vi "Draw Trajectory.vi"(0 "Picture in":refnum<vi>, 1 "Robot Index":i32, 5 "Trajectory Data":T3, 7 "time":dbl, 9 "new picture in":picture, 10 "MEGA?":bool, 11 "Hide Path":bool, 12 "MEGA traj":T2 {"?"."Limits"."StoopidFast (fps)" min=0.0; "?"."Limits"."Jerk (fps^3)" min=0.0 step=1.0; "?"."Limits"."Accel (fps^2)" min=0.0; "?"."Limits"."Velocity (fps)" min=0.0; "?"."Overrides"."Angle Override" step=5.0; "?"."Overrides"."Velocity Override" step=5.0; "?"."Overrides"."Angular Override" step=5.0; "?"."Angular Limits"."Jerk (deg/s^3)" min=0.0 step=1.0; "?"."Angular Limits"."Accel (deg/s^2)" min=0.0; "?"."Angular Limits"."Velocity (deg/s)" min=0.0}) -> (3 "Path Points MEGA":cluster{"x":dbl, "y":dbl}[][](array[cluster]), 4 "new picture":picture, 6 "Output Point":T12, 14 "Output Point MEGA":T1(array[cluster]), 15 "Path Points":cluster{"x":dbl, "y":dbl}[](array[cluster]))   [LabVIEW 2023]
uses:
  Types/Trajectory Data.ctl
  Types/Segment Type.ctl
  FileIO/MEGA traj.ctl
  Types/Single Cmd Info.ctl
  <vilib>/picture/picture.llb/imagedata.ctl
  Types/Limits.ctl
  Types/Overrides.ctl
  Types/Angluar Limits.ctl
  Types/Drive Type.ctl
  Types/Path Type.ctl
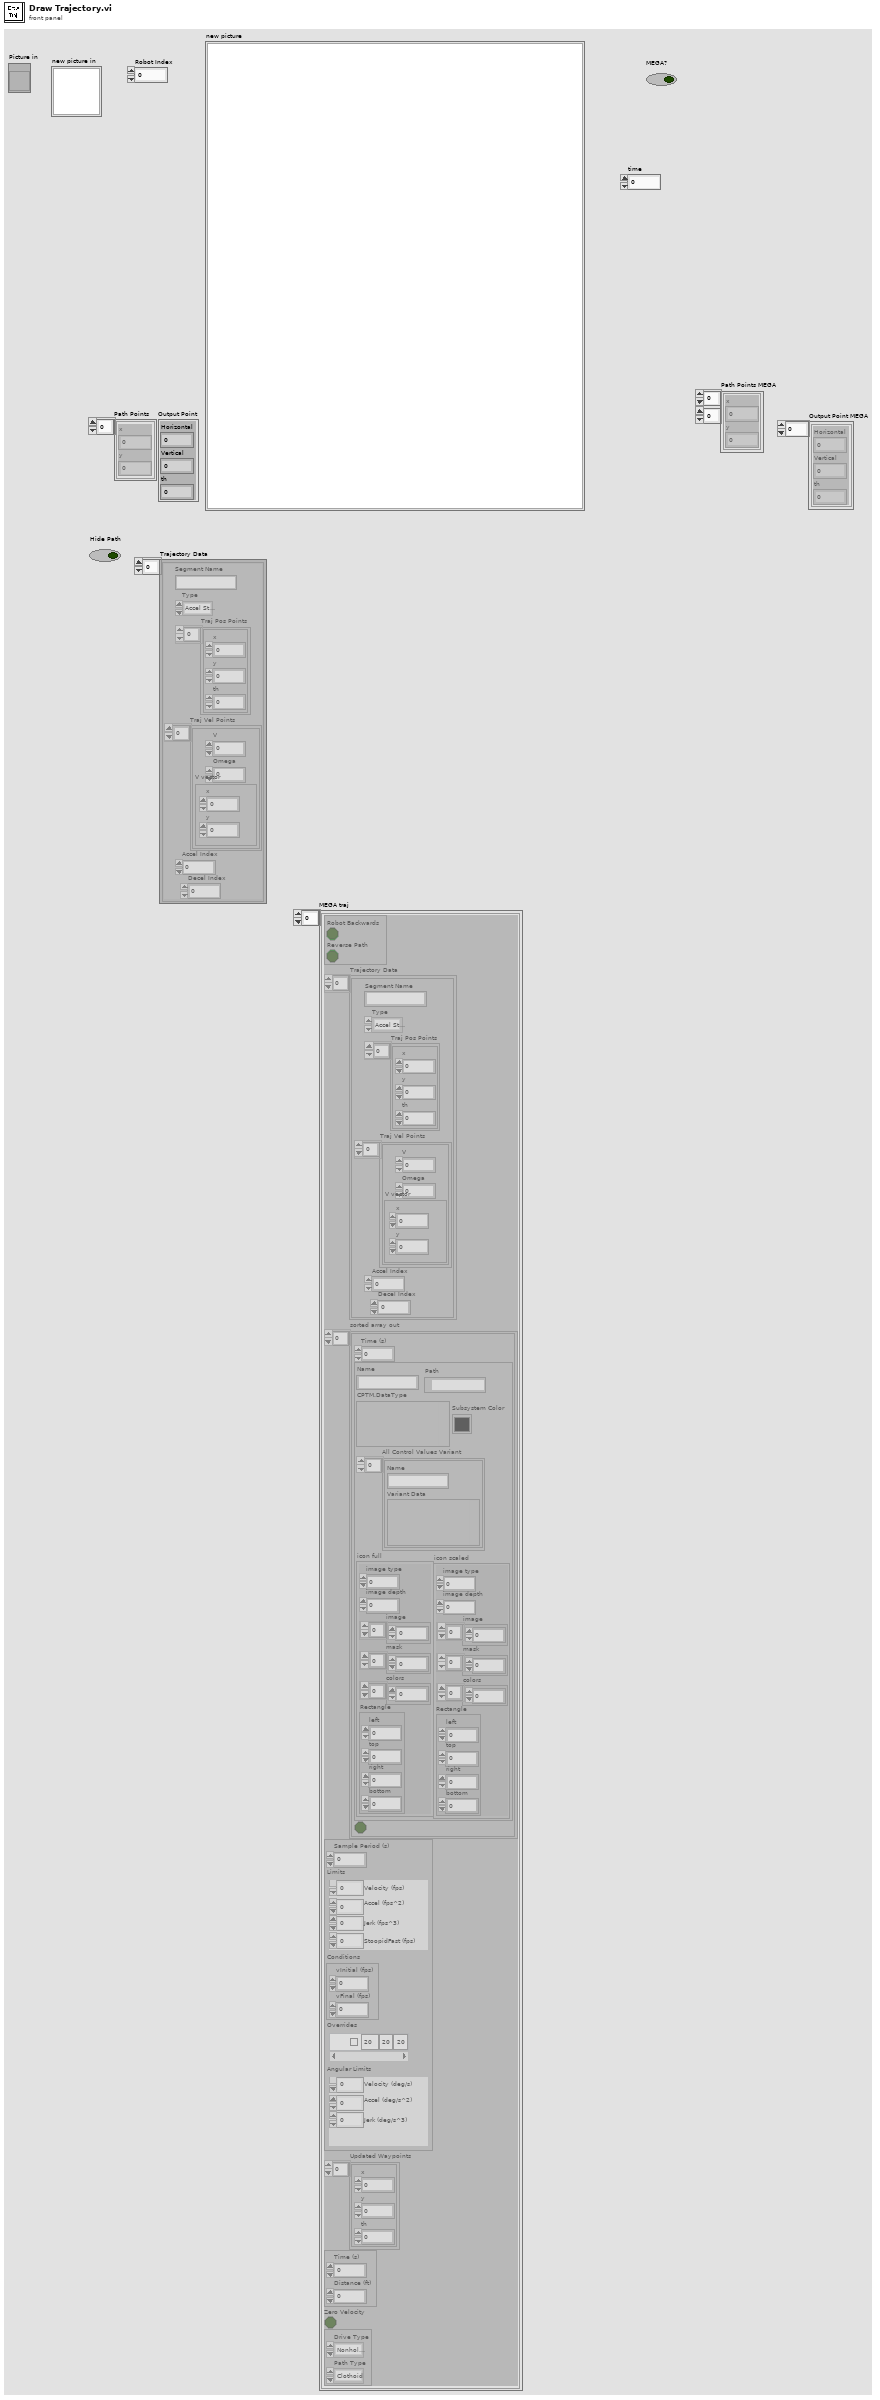
[diagram p1: front panel]
types:
  T1 = cluster{"Horizontal":dbl, "Vertical":dbl, "th":dbl}[]
  T2 = typedef "MEGA traj.ctl" = cluster{cluster{"Robot Backwards":bool, "Reverse Path":bool}, "Trajectory Data":T3, "sorted array out":cluster{"Time (s)":dbl, T5, bool}[], cluster{"Sample Period (s)":dbl, "Limits":T7, "Conditions":cluster{"vInitial (fps)":dbl, "vFinal (fps)":dbl}, "Overrides":T8, "Angular Limits":T9}, "Updated Waypoints":cluster{"x":dbl, "y":dbl, "th":dbl}[], cluster{"Time (s)":dbl, "Distance (ft)":dbl}, "Zero Velocity":bool, cluster{"Drive Type":T10, "Path Type":T11}}[]
  T3 = typedef "Trajectory Data.ctl" = cluster{"Segment Name":string, "Type":T4, "Traj Pos Points":cluster{"x":dbl, "y":dbl, "th":dbl}[], "Traj Vel Points":cluster{"V":dbl, "Omega":dbl, "V vector":cluster{"y":dbl, "x":dbl}}[], "Accel Index":i32, "Decel Index":i32}[]
  T4 = typedef "Segment Type.ctl" = enum16{"Accel Straight", "Const Straight", "Blend", "Circle", "Bezier"}
  T5 = typedef "Single Cmd Info.ctl" = cluster{"Name":string, "CPTM.DataType":variant, "All Control Values Variant":cluster{"Name":string, "Variant Data":variant}[], "icon full":T6, "icon scaled":T6, "Path":path, "Subsystem Color":u32}
  T6 = typedef "imagedata.ctl" = cluster{"image type":i32, "image depth":i32, "image":u8[], "mask":u8[], "colors":u32[], "Rectangle":cluster{"left":i16, "top":i16, "right":i16, "bottom":i16}}
  T7 = typedef "Limits.ctl" = cluster{"Velocity (fps)":dbl, "Accel (fps^2)":dbl, "Jerk (fps^3)":dbl, "StoopidFast (fps)":dbl}
  T8 = typedef "Overrides.ctl" = cluster{"Count":string, "Angular Override":dbl, "Enabled?":bool, "Velocity Override":dbl, "Angle Override":dbl}[]
  T9 = typedef "Angluar Limits.ctl" = cluster{"Velocity (deg/s)":dbl, "Accel (deg/s^2)":dbl, "Jerk (deg/s^3)":dbl}
  T10 = typedef "Drive Type.ctl" = enum16{"Nonholonomic", "Holonomic"}
  T11 = typedef "Path Type.ctl" = enum16{"Clothoid", "Bezier"}
  T12 = cluster{"Horizontal":dbl, "Vertical":dbl, "th":dbl}
  T13 = cluster{"Width":u16, "Style":enum32{"Solid", "Dash", "Dot", "DashDot", "DashDotDot"}}
  T14 = typedef "LVPositionTypeDef.ctl" = cluster{"Left":i32, "Top":i32}
  T15 = typedef "LVBoundsTypeDef.ctl" = cluster{"Width":u32, "Height":u32}
  T16 = cluster{"V":dbl, "Omega":dbl, "V vector":cluster{"y":dbl, "x":dbl}}[]
  T17 = cluster{cluster{"Robot Backwards":bool, "Reverse Path":bool}, "Trajectory Data":T3, "sorted array out":cluster{"Time (s)":dbl, T5, bool}[], cluster{"Sample Period (s)":dbl, "Limits":T7, "Conditions":cluster{"vInitial (fps)":dbl, "vFinal (fps)":dbl}, "Overrides":T8, "Angular Limits":T9}, "Updated Waypoints":cluster{"x":dbl, "y":dbl, "th":dbl}[], cluster{"Time (s)":dbl, "Distance (ft)":dbl}, "Zero Velocity":bool, cluster{"Drive Type":T10, "Path Type":T11}}
  T18 = cluster{"Robot Backwards":bool, "Reverse Path":bool}
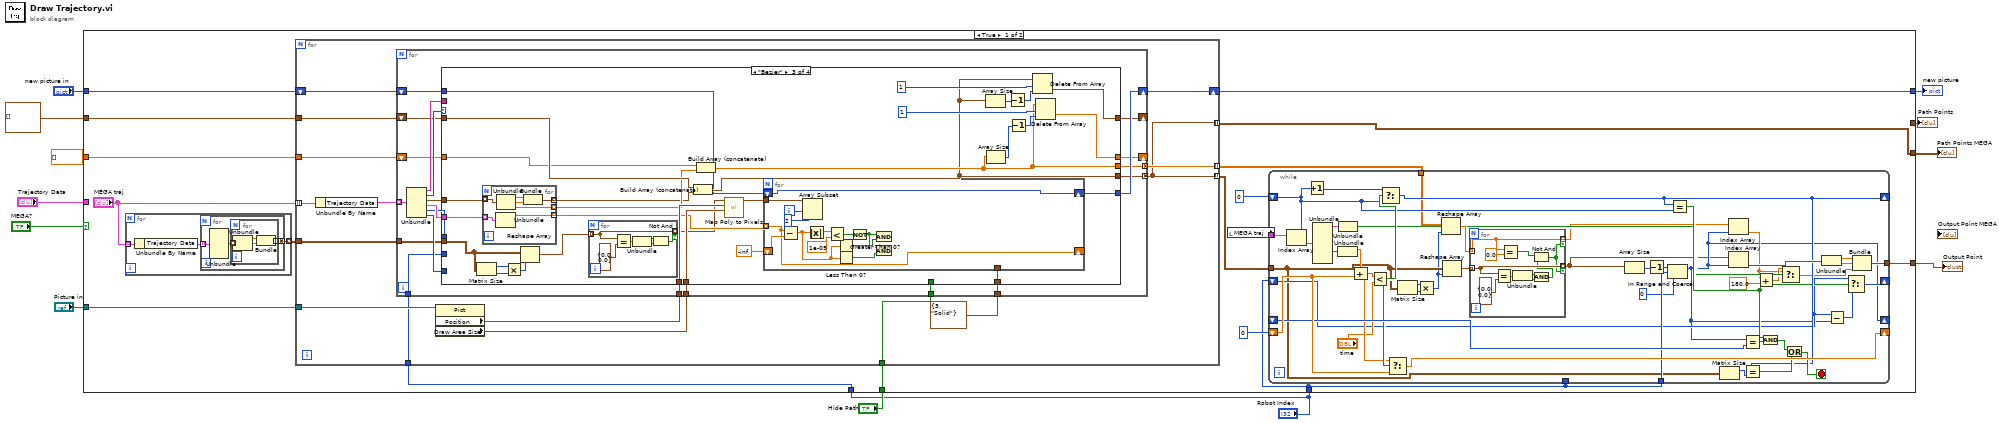
[diagram p0: block diagram]
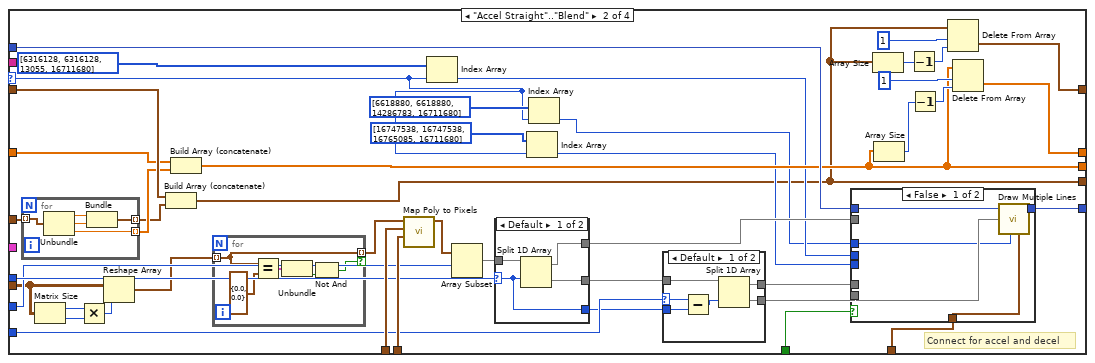
[diagram p3: hidden frame]
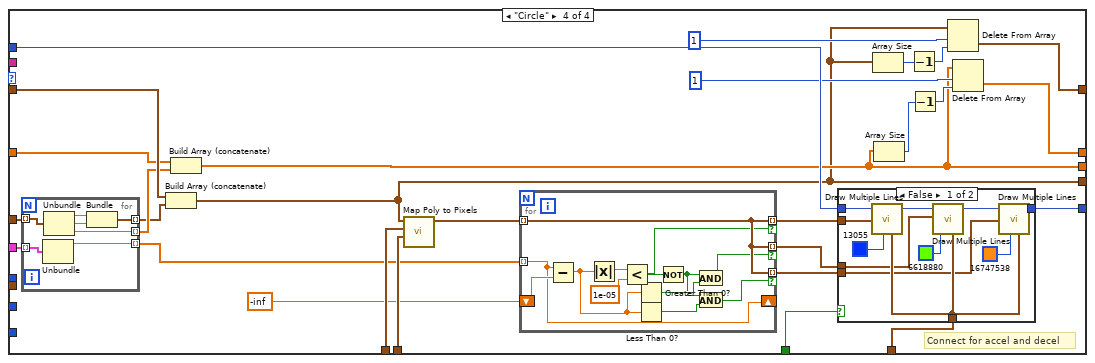
[diagram p7: hidden frame]
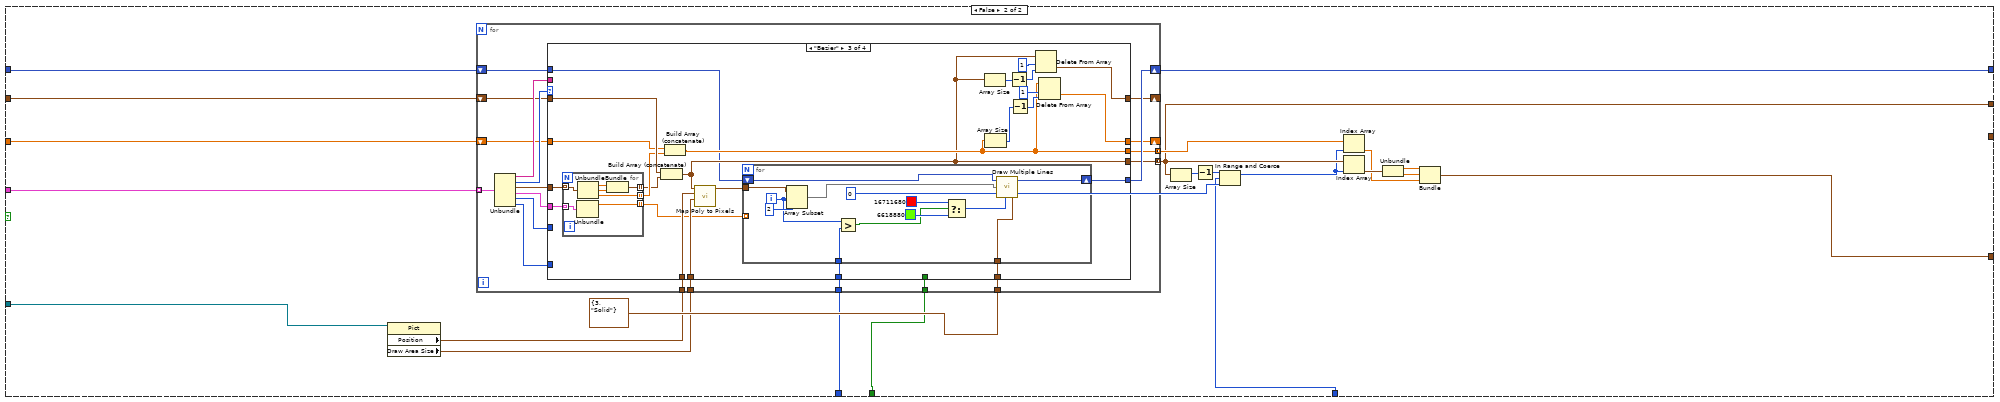
[diagram p9: hidden frame]
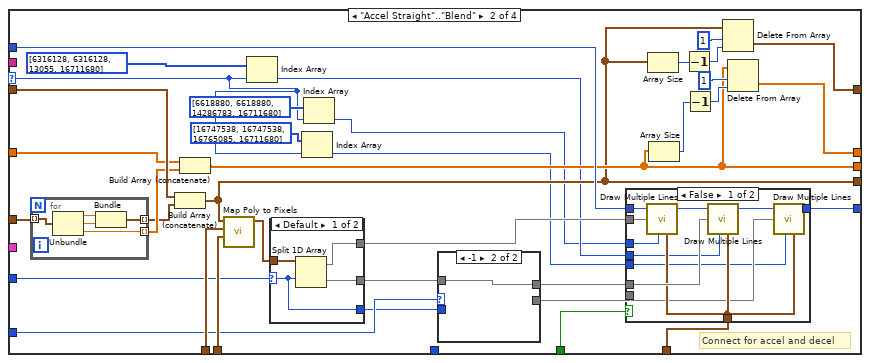
[diagram p11: hidden frame]
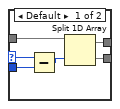
[diagram p13: hidden frame]
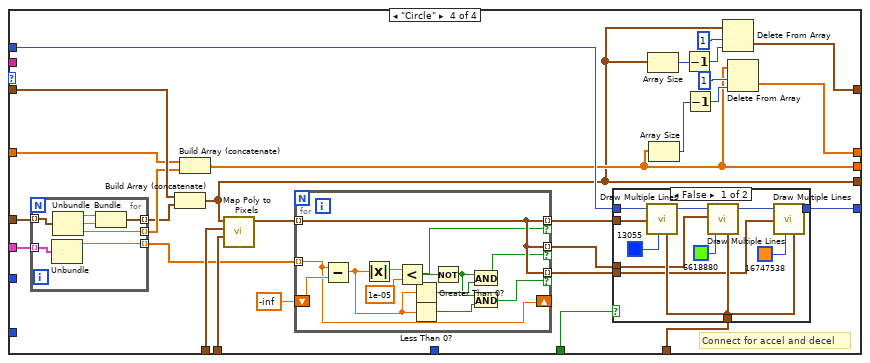
[diagram p15: hidden frame]
diagram:
  n1 = case shown="True" "MEGA?" {
    tunnel: "Picture in" -> [w29 w345]
    tunnel: "new picture in" -> [w28 w344]
    tunnel: [w27 w340] -> w10
    tunnel: [_ w334] -> w9
    tunnel: cluster{"x":dbl, "y":dbl}[] [] -> [w26 w329]
    tunnel: dbl[] [] -> [w25 w328]
    tunnel: "Trajectory Data" -> [_ w327]
    tunnel: "Hide Path" -> [w24 w326]
    tunnel: [w17 _] -> w3
    tunnel: "Robot Index" -> [w16 w325]
    tunnel: [w21 w324] -> w2
    tunnel: "Robot Index" -> [w15 w323]
    frame True {
      n2 = for {
        tunnel: "MEGA traj" -> [w32] mode=indexing
        tunnel: [w30] -> w13 mode=indexing
        n3 = Unbundle By Name(w32) -> ("Trajectory Data"=w31:T3)
        n4 = for {
          tunnel: w31 -> [w35] mode=indexing
          tunnel: [w33] -> w30 mode=concatenating
          n5 = Unbundle(w35) -> ("Traj Pos Points"=w34:cluster{"x":dbl, "y":dbl, "th":dbl}[])  [unwired: 5 out]
          n6 = for {
            tunnel: w34 -> [w37] mode=indexing
            tunnel: [w36] -> w33 mode=indexing
            n7 = Unbundle(w37) -> ("x"=w39:dbl, "y"=w38:dbl)  [unwired: 1 out]
            n8 = Bundle("x"=w39, "y"=w38) -> (w36:cluster{"x":dbl, "y":dbl})  [unwired: 1 in]
          }
        }
      }
      n9 = for {
        tunnel: w29 -> [w110]
        tunnel: [w99] -> w17 mode=indexing
        tunnel: w26 -> [w104]
        tunnel: w25 -> [w103]
        shift-right: [w105] -> w27
        shift-left: w28 -> [w109]
        tunnel: w24 -> [w102]
        tunnel: "MEGA traj" -> [w97] mode=indexing
        tunnel: [w100] -> w18 mode=indexing
        tunnel: [w99] -> w19 mode=indexing
        tunnel: w15 -> [w98]
        tunnel: w13 -> [w96]
        n10 = Unbundle By Name(w97) -> ("Trajectory Data"=w101:T3)
        n11 = property on="Property Node" class="Pict"(reference=w110) -> ("Position"=w106:T14, "Draw Area Size"=w107:T15)  [unwired: 1 in, 2 out]
        n12 = for {
          tunnel: w101 -> [w131] mode=indexing
          shift-right: [w125] -> w105
          shift-left: w109 -> [w124]
          tunnel: T13 {"Width"=3, "Style"=enum."Solid"} ("pen") -> [w128]
          tunnel: w107 -> [w127]
          tunnel: w106 -> [w126]
          tunnel: [w122] -> w99 mode=concatenating
          tunnel: [w121] -> w100 mode=concatenating
          shift-right: [w120] -> _
          shift-left: w104 -> [w119]
          shift-right: [w118] -> _
          shift-left: w103 -> [w117]
          tunnel: w102 -> [w115]
          tunnel: w98 -> [w112]
          tunnel: w96 -> [w111]
          n13 = Unbundle(w131) -> ("Segment Name"=w130:string, "Type"=w123:T4, "Traj Pos Points"=w113:cluster{"x":dbl, "y":dbl, "th":dbl}[], "Traj Vel Points"=w129:T16, "Accel Index"=w114:i32, "Decel Index"=w116:i32)
          n14 = case shown="\"Bezier\"" w123 {
            selector: w123 -> [_ w148 _ _]
            tunnel: w130 -> [_ _ _ _]
            tunnel: w113 -> [_ w178 w237 w291]
            tunnel: w129 -> [_ _ w220 w270]
            tunnel: w128 -> [_ w157 w217 w274]
            tunnel: w127 -> [_ w177 w236 w290]
            tunnel: w126 -> [_ w175 w235 w288]
            tunnel: [w134 w158 w215 w275] -> w125
            tunnel: w124 -> [w134 w176 w216 w289]
            tunnel: [_ w142 w221 w272] -> w122
            tunnel: [_ w164 w225 w278] -> w121
            tunnel: w114 -> [_ w161 _ _]
            tunnel: [w133 w169 w230 w283] -> w120
            tunnel: w119 -> [w133 w172 w233 w286]
            tunnel: [w132 w165 w226 w279] -> w118
            tunnel: w117 -> [w132 w162 w223 w276]
            tunnel: w116 -> [_ w160 _ _]
            tunnel: w115 -> [_ w145 _ w271]
            tunnel: w112 -> [_ w141 _ _]
            tunnel: w111 -> [_ w140 w210 _]
            frame Default {
            }
            frame "Accel Straight".."Blend" {
              # "Connect for accel and decel"
              n15 = for {
                tunnel: w178 -> [w207] mode=indexing
                tunnel: [w206] -> w153 mode=indexing
                tunnel: [w203] -> w163 mode=indexing
                n16 = Unbundle(w207) -> ("x"=w205:dbl, "y"=w204:dbl, "th"=w203:dbl)
                n17 = Bundle("x"=w205, "y"=w204) -> (w206:cluster{"x":dbl, "y":dbl})  [unwired: 1 in]
              }
              n18 = Matrix Size(0:w140) -> (1:w139:i32, 2:w138:i32)
              n19 = Multiply(x=w139, y=w138) -> (x*y=w137:i32)
              n20 = Reshape Array(w140, w137) -> (w136:cluster{"x":dbl, "y":dbl}[])
              n21 = Build Array (concatenate)(w172, w153) -> (w142:cluster{"x":dbl, "y":dbl}[])
              n22 = Build Array (concatenate)(w162, w163) -> (w164:dbl[])
              n23 = for {
                tunnel: w136 -> [w184] mode=indexing
                tunnel: [w184] -> w135 mode=indexing if=w179
                n24 = Equal?(x=w184, y=cluster{"x":dbl, "y":dbl} {"x"=0.0, "y"=0.0}) -> (x = y?=w182:cluster{"x":bool, "y":bool})
                n25 = Unbundle(w182) -> ("x"=w180:bool, "y"=w181:bool)
                n26 = Not And(1:w181, 2:w180) -> (0:w179:bool)
              }
              n27 = call "Map Poly to Pixels.vi"("Draw Area Size"=w177, "Position"=w175, "Coords"=w135) -> ("Coords"=w143:cluster{"Horizontal":dbl, "Vertical":dbl}[])  [unwired: 8 in]
              n28 = Index Array(array=u32[] [6316128, 6316128, 13055, 16711680], index=w148) -> (element=w151:u32)
              n29 = Array Subset(array=w143, index=w141) -> (w144:cluster{"Horizontal":dbl, "Vertical":dbl}[])  [unwired: 1 in]
              n30 = case shown="Default" w161 {
                selector: w161 -> [w198 _]
                tunnel: w144 -> [w201 w202]
                tunnel: [w199 _] -> w152
                tunnel: [w200 w202] -> w155
                tunnel: [w198 _] -> w154
                frame Default {
                  n31 = Split 1D Array(array=w201, index=w198) -> (first subarray=w199:cluster{"Horizontal":dbl, "Vertical":dbl}[], second subarray=w200:cluster{"Horizontal":dbl, "Vertical":dbl}[])
                }
                frame -1 {
                }
              }
              n32 = Index Array(array=u32[] [16747538, 16747538, 16765085, 16711680], index=w148) -> (element=w146:u32)
              n33 = Index Array(array=u32[] [6618880, 6618880, 14286783, 16711680], index=w148) -> (element=w147:u32)
              n34 = case shown="Default" w160 {
                selector: w160 -> [w193 _]
                tunnel: w155 -> [w196 w197]
                tunnel: [w195 w197] -> w159
                tunnel: [w194 _] -> w156
                tunnel: w154 -> [w192 _]
                frame Default {
                  n35 = Subtract(x=w193, y=w192) -> (x-y=w191:i32)
                  n36 = Split 1D Array(array=w196, index=w191) -> (first subarray=w195:cluster{"Horizontal":dbl, "Vertical":dbl}[], second subarray=w194:cluster{"Horizontal":dbl, "Vertical":dbl}[])
                }
                frame -1 {
                }
              }
              n37 = case shown="False" w145 {
                tunnel: w176 -> [w186 w190]
                tunnel: w159 -> [_ _]
                tunnel: [w189 w190] -> w158
                tunnel: w157 -> [w188 _]
                tunnel: w156 -> [w187 _]
                tunnel: w152 -> [_ _]
                tunnel: w151 -> [_ _]
                tunnel: w147 -> [w185 _]
                tunnel: w146 -> [_ _]
                frame False {
                  n38 = call <vilib>:"Draw Multiple Lines.vi"("picture"=w186, "line endpoints"=w187, "color(black)"=w185, "pen"=w188) -> ("new picture"=w189:picture)  [unwired: 5 in]
                }
                frame True {
                }
              }
              n39 = Array Size(array=w142) -> (size(s)=w173:i32)
              n40 = Array Size(array=w164) -> (size(s)=w166:i32)
              n41 = Decrement(x=w173) -> (x-1=w170:i32)
              n42 = Decrement(x=w166) -> (x-1=w168:i32)
              n43 = Delete From Array(array=w142, length=1, index=w170) -> (deleted portion=w169:cluster{"x":dbl, "y":dbl}[])  [unwired: 1 out]
              n44 = Delete From Array(array=w164, length=1, index=w168) -> (deleted portion=w165:dbl[])  [unwired: 1 out]
            }
            frame "Bezier" {
              n45 = Matrix Size(0:w210) -> (1:w209:i32, 2:w213:i32)
              n46 = for {
                tunnel: w237 -> [w263] mode=indexing
                tunnel: [w262] -> w222 mode=indexing
                tunnel: [w259] -> w224 mode=indexing
                tunnel: w220 -> [w258] mode=indexing
                tunnel: [w257] -> w219 mode=indexing
                n47 = Unbundle(w258) -> ("V"=w257:dbl)  [unwired: 2 out]
                n48 = Unbundle(w263) -> ("x"=w261:dbl, "y"=w260:dbl, "th"=w259:dbl)
                n49 = Bundle("x"=w261, "y"=w260) -> (w262:cluster{"x":dbl, "y":dbl})  [unwired: 1 in]
              }
              n50 = Multiply(x=w209, y=w213) -> (x*y=w212:i32)
              n51 = Reshape Array(w210, w212) -> (w211:cluster{"x":dbl, "y":dbl}[])
              n52 = for {
                tunnel: w211 -> [w243] mode=indexing
                tunnel: [w243] -> w208 mode=indexing if=w238
                n53 = Equal?(x=w243, y=cluster{"x":dbl, "y":dbl} {"x"=0.0, "y"=0.0}) -> (x = y?=w241:cluster{"x":bool, "y":bool})
                n54 = Unbundle(w241) -> ("x"=w239:bool, "y"=w240:bool)
                n55 = Not And(1:w240, 2:w239) -> (0:w238:bool)
              }
              n56 = Build Array (concatenate)(w233, w222) -> (w221:cluster{"x":dbl, "y":dbl}[])
              n57 = Build Array (concatenate)(w223, w224) -> (w225:dbl[])
              n58 = call "Map Poly to Pixels.vi"("Draw Area Size"=w236, "Position"=w235, "Coords"=w208) -> ("Coords"=w214:cluster{"Horizontal":dbl, "Vertical":dbl}[])  [unwired: 8 in]
              n59 = for {
                tunnel: w214 -> [w245]
                tunnel: w219 -> [w253] mode=indexing
                shift-right: [w253] -> _
                shift-left: -inf -> [w256]
                tunnel: w217 -> [_]
                shift-right: [w244] -> w215
                shift-left: w216 -> [w244]
                i -> [w247]
                n60 = Subtract(x=w253, y=w256) -> (x-y=w251:dbl)
                n61 = Array Subset(array=w245, index=w247, length=2) -> ()  [unwired: 1 out]
                n62 = Absolute Value(x=w251) -> (abs(x)=w255:dbl)
                n63 = Less?(x=w255, y=1e-05) -> (x < y?=w248:bool)
                n64 = Greater Than 0?(x=w251) -> (x > 0?=w252:bool)
                n65 = Less Than 0?(x=w251) -> (x < 0?=w250:bool)
                n66 = Not(x=w248) -> (.not. x?=w249:bool)
                n67 = And(x=w249, y=w252) -> ()  [unwired: 1 out]
                n68 = And(x=w249, y=w250) -> ()  [unwired: 1 out]
              }
              n69 = Array Size(array=w221) -> (size(s)=w234:i32)
              n70 = Array Size(array=w225) -> (size(s)=w227:i32)
              n71 = Decrement(x=w234) -> (x-1=w231:i32)
              n72 = Decrement(x=w227) -> (x-1=w229:i32)
              n73 = Delete From Array(array=w221, length=1, index=w231) -> (deleted portion=w230:cluster{"x":dbl, "y":dbl}[])  [unwired: 1 out]
              n74 = Delete From Array(array=w225, length=1, index=w229) -> (deleted portion=w226:dbl[])  [unwired: 1 out]
            }
            frame "Circle" {
              # "Connect for accel and decel"
              n75 = for {
                tunnel: w291 -> [w322] mode=indexing
                tunnel: [w321] -> w273 mode=indexing
                tunnel: [w318] -> w277 mode=indexing
                tunnel: w270 -> [w317] mode=indexing
                tunnel: [w316] -> w269 mode=indexing
                n76 = Unbundle(w317) -> ("V"=w316:dbl)  [unwired: 2 out]
                n77 = Unbundle(w322) -> ("x"=w320:dbl, "y"=w319:dbl, "th"=w318:dbl)
                n78 = Bundle("x"=w320, "y"=w319) -> (w321:cluster{"x":dbl, "y":dbl})  [unwired: 1 in]
              }
              n79 = Build Array (concatenate)(w286, w273) -> (w272:cluster{"x":dbl, "y":dbl}[])
              n80 = Build Array (concatenate)(w276, w277) -> (w278:dbl[])
              n81 = call "Map Poly to Pixels.vi"("Draw Area Size"=w290, "Position"=w288, "Coords"=w272) -> ("Coords"=w264:cluster{"Horizontal":dbl, "Vertical":dbl}[])  [unwired: 8 in]
              n82 = for {
                tunnel: w264 -> [w300] mode=indexing
                tunnel: w269 -> [w299] mode=indexing
                shift-right: [w299] -> _
                shift-left: -inf -> [w303]
                tunnel: [w300] -> w267 mode=indexing if=w294
                tunnel: [w300] -> w266 mode=indexing if=w293
                tunnel: [w300] -> w265 mode=indexing if=w292
                n83 = Subtract(x=w299, y=w303) -> (x-y=w297:dbl)
                n84 = Absolute Value(x=w297) -> (abs(x)=w302:dbl)
                n85 = Less?(x=w302, y=1e-05) -> (x < y?=w294:bool)
                n86 = Greater Than 0?(x=w297) -> (x > 0?=w298:bool)
                n87 = Less Than 0?(x=w297) -> (x < 0?=w296:bool)
                n88 = Not(x=w294) -> (.not. x?=w295:bool)
                n89 = And(x=w295, y=w298) -> (x .and. y?=w293:bool)
                n90 = And(x=w295, y=w296) -> (x .and. y?=w292:bool)
              }
              n91 = case shown="False" w271 {
                tunnel: w289 -> [w314 w315]
                tunnel: [w311 w315] -> w275
                tunnel: w274 -> [w310 _]
                tunnel: w267 -> [w307 _]
                tunnel: w266 -> [w306 _]
                tunnel: w265 -> [w305 _]
                frame False {
                  n92 = call <vilib>:"Draw Multiple Lines.vi"("picture"=w314, "line endpoints"=w307, "color(black)"=u32 13055, "pen"=w310) -> ("new picture"=w313:picture)  [unwired: 5 in]
                  n93 = call <vilib>:"Draw Multiple Lines.vi"("picture"=w313, "line endpoints"=w306, "color(black)"=u32 6618880, "pen"=w310) -> ("new picture"=w312:picture)  [unwired: 5 in]
                  n94 = call <vilib>:"Draw Multiple Lines.vi"("picture"=w312, "line endpoints"=w305, "color(black)"=u32 16747538, "pen"=w310) -> ("new picture"=w311:picture)  [unwired: 5 in]
                }
                frame True {
                }
              }
              n95 = Array Size(array=w272) -> (size(s)=w287:i32)
              n96 = Array Size(array=w278) -> (size(s)=w280:i32)
              n97 = Decrement(x=w287) -> (x-1=w284:i32)
              n98 = Decrement(x=w280) -> (x-1=w282:i32)
              n99 = Delete From Array(array=w272, length=1, index=w284) -> (deleted portion=w283:cluster{"x":dbl, "y":dbl}[])  [unwired: 1 out]
              n100 = Delete From Array(array=w278, length=1, index=w282) -> (deleted portion=w279:dbl[])  [unwired: 1 out]
            }
          }
        }
      }
      n101 = local read "MEGA traj"() -> (w23:T2)
      n102 = while {
        tunnel: w16 -> [w61]
        tunnel: w19 -> [w56]
        tunnel: w18 -> [w57]
        shift-right: [w66] -> _
        shift-left: 0 -> [w65]
        tunnel: w23 -> [w84]
        shift-right: [w79] -> _
        shift-left: 0 -> [w80]
        shift-right: [w42] -> _
        shift-left: _ -> [w72]
        shift-right: [w64] -> _
        shift-left: w16 -> [w60]
        tunnel: [w50] -> w21
        tunnel: w16 -> [_]
        stop <- w73 stop-if-true
        n103 = Index Array(array=w84, index=w65) -> (element=w83:T17)
        n104 = Increment(x=w65) -> (x+1=w85:i32)
        n105 = Unbundle(w83) -> (w48:T18, w82:cluster{"Time (s)":dbl, "Distance (ft)":dbl})  [unwired: 6 out]
        n106 = Unbundle(w82) -> ("Time (s)"=w81:dbl)  [unwired: 1 out]
        n107 = Unbundle(w48) -> ("Robot Backwards"=w47:bool)  [unwired: 1 out]
        n108 = Add(x=w81, y=w80) -> (x+y=w70:dbl)
        n109 = Less?(x=w70, y="time") -> (x < y?=w71:bool)
        n110 = Select(t=w85, s=w71, f=w65) -> (s? t:f=w66:i32)
        n111 = Select(t=w70, s=w71, f=w80) -> (s? t:f=w79:dbl)
        n112 = Matrix Size(0:w56) -> (1:w55:i32, 2:w54:i32)
        n113 = Multiply(x=w55, y=w54) -> (x*y=w53:i32)
        n114 = Reshape Array(w57, w53) -> (w51:dbl[])
        n115 = Reshape Array(w56, w53) -> (w52:cluster{"x":dbl, "y":dbl}[])
        n116 = for {
          tunnel: w52 -> [w95] mode=indexing
          tunnel: [w95] -> w40 mode=indexing if=w88
          tunnel: w51 -> [w92] mode=indexing
          tunnel: [w92] -> w41 mode=indexing if=w88
          n117 = Equal?(x=w95, y=cluster{"x":dbl, "y":dbl} {"x"=0.0, "y"=0.0}) -> (x = y?=w93:cluster{"x":bool, "y":bool})
          n118 = Equal?(x=w92, y=0.0) -> (x = y?=w86:bool)
          n119 = Unbundle(w93) -> ("x"=w89:bool, "y"=w90:bool)
          n120 = And(x=w89, y=w90) -> (x .and. y?=w87:bool)
          n121 = Not And(1:w87, 2:w86) -> (0:w88:bool)
        }
        n122 = Array Size(array=w40) -> (size(s)=w58:i32)
        n123 = Decrement(x=w58) -> (x-1=w59:i32)
        n124 = In Range and Coerce(upper limit=w59, x=w61, lower limit=u16 0 ("Width")) -> (coerced(x)=w42:i32)  [unwired: 1 out]
        n125 = Equal?(x=w66, y=w65) -> (x = y?=w63:bool)
        n126 = Matrix Size(0:w56) -> (1:w75:i32)  [unwired: 1 out]
        n127 = Index Array(array=w41, index=w42) -> (element=w44:dbl)
        n128 = Index Array(array=w40, index=w42) -> (element=w78:cluster{"x":dbl, "y":dbl})
        n129 = Equal?(x=w42, y=w72) -> (x = y?=w68:bool)
        n130 = Equal?(x=w66, y=w75) -> (x = y?=w74:bool)
        n131 = Add(x=w44, y=180.0) -> (x+y=w45:dbl)
        n132 = And(x=w63, y=w68) -> (x .and. y?=w67:bool)
        n133 = Select(t=w45, s=w47, f=w44) -> (s? t:f=w46:dbl)
        n134 = Or(x=w67, y=w74) -> (x .or. y?=w73:bool)
        n135 = Unbundle(w78) -> ("x"=w77:dbl, "y"=w76:dbl)
        n136 = Subtract(x=w60, y=w42) -> (x-y=w62:i32)
        n137 = Select(t=w60, s=w63, f=w62) -> (s? t:f=w64:i32)
        n138 = Bundle("x"=w77, "y"=w76, "th"=w46) -> (w50:cluster{"x":dbl, "y":dbl, "th":dbl})  [unwired: 1 in]
      }
    }
    frame False {
      n139 = property on="Property Node" class="Pict"(reference=w345) -> ("Position"=w341:T14, "Draw Area Size"=w342:T15)  [unwired: 1 in, 2 out]
      n140 = for {
        tunnel: w327 -> [w365] mode=indexing
        shift-right: [w358] -> w340
        shift-left: w344 -> [w357]
        tunnel: T13 {"Width"=3, "Style"=enum."Solid"} ("pen") -> [w361]
        tunnel: w342 -> [w360]
        tunnel: w341 -> [w359]
        tunnel: [w355] -> w334 mode=concatenating
        tunnel: [w354] -> w335 mode=concatenating
        shift-right: [w352] -> _
        shift-left: w329 -> [w351]
        shift-right: [w350] -> _
        shift-left: w328 -> [w349]
        tunnel: w326 -> [w347]
        tunnel: w323 -> [w346]
        n141 = Unbundle(w365) -> ("Segment Name"=w364:string, "Type"=w356:T4, "Traj Pos Points"=w363:cluster{"x":dbl, "y":dbl, "th":dbl}[], "Traj Vel Points"=w362:T16, "Accel Index"=w353:i32, "Decel Index"=w348:i32)
        n142 = case shown="\"Bezier\"" w356 {
          selector: w356 -> [_ w372 _ _]
          tunnel: w364 -> [_ _ _ _]
          tunnel: w363 -> [_ w404 w457 w504]
          tunnel: w362 -> [_ _ w440 w483]
          tunnel: w361 -> [_ w383 w435 w487]
          tunnel: w360 -> [_ w403 w456 w503]
          tunnel: w359 -> [_ w401 w455 w501]
          tunnel: [w368 w384 w436 w488] -> w358
          tunnel: w357 -> [w368 w402 w437 w502]
          tunnel: [_ w378 w441 w485] -> w355
          tunnel: [_ w390 w445 w491] -> w354
          tunnel: w353 -> [_ w387 _ _]
          tunnel: [w367 w395 w450 w496] -> w352
          tunnel: w351 -> [w367 w398 w453 w499]
          tunnel: [w366 w391 w446 w492] -> w350
          tunnel: w349 -> [w366 w388 w443 w489]
          tunnel: w348 -> [_ w386 _ _]
          tunnel: w347 -> [_ w369 _ w484]
          tunnel: w346 -> [_ _ w434 _]
          frame Default {
          }
          frame "Accel Straight".."Blend" {
            # "Connect for accel and decel"
            n143 = for {
              tunnel: w404 -> [w433] mode=indexing
              tunnel: [w432] -> w379 mode=indexing
              tunnel: [w429] -> w389 mode=indexing
              n144 = Unbundle(w433) -> ("x"=w431:dbl, "y"=w430:dbl, "th"=w429:dbl)
              n145 = Bundle("x"=w431, "y"=w430) -> (w432:cluster{"x":dbl, "y":dbl})  [unwired: 1 in]
            }
            n146 = Build Array (concatenate)(w398, w379) -> (w378:cluster{"x":dbl, "y":dbl}[])
            n147 = Build Array (concatenate)(w388, w389) -> (w390:dbl[])
            n148 = call "Map Poly to Pixels.vi"("Draw Area Size"=w403, "Position"=w401, "Coords"=w378) -> ("Coords"=w377:cluster{"Horizontal":dbl, "Vertical":dbl}[])  [unwired: 8 in]
            n149 = Index Array(array=u32[] [6316128, 6316128, 13055, 16711680], index=w372) -> (element=w375:u32)
            n150 = case shown="Default" w387 {
              selector: w387 -> [w424 _]
              tunnel: w377 -> [w427 w428]
              tunnel: [w425 _] -> w376
              tunnel: [w426 w428] -> w381
              tunnel: [w424 _] -> w380
              frame Default {
                n151 = Split 1D Array(array=w427, index=w424) -> (first subarray=w425:cluster{"Horizontal":dbl, "Vertical":dbl}[], second subarray=w426:cluster{"Horizontal":dbl, "Vertical":dbl}[])
              }
              frame -1 {
              }
            }
            n152 = Index Array(array=u32[] [16747538, 16747538, 16765085, 16711680], index=w372) -> (element=w370:u32)
            n153 = Index Array(array=u32[] [6618880, 6618880, 14286783, 16711680], index=w372) -> (element=w371:u32)
            n154 = case shown="-1" w386 {
              selector: w386 -> [w419 _]
              tunnel: w381 -> [w422 w423]
              tunnel: [w421 w423] -> w385
              tunnel: [w420 _] -> w382
              tunnel: w380 -> [w418 _]
              frame Default {
                n155 = Subtract(x=w419, y=w418) -> (x-y=w417:i32)
                n156 = Split 1D Array(array=w422, index=w417) -> (first subarray=w421:cluster{"Horizontal":dbl, "Vertical":dbl}[], second subarray=w420:cluster{"Horizontal":dbl, "Vertical":dbl}[])
              }
              frame -1 {
              }
            }
            n157 = case shown="False" w369 {
              tunnel: w402 -> [w415 w416]
              tunnel: w385 -> [w413 _]
              tunnel: [w411 w416] -> w384
              tunnel: w383 -> [w410 _]
              tunnel: w382 -> [w409 _]
              tunnel: w376 -> [w408 _]
              tunnel: w375 -> [w407 _]
              tunnel: w371 -> [w406 _]
              tunnel: w370 -> [w405 _]
              frame False {
                n158 = call <vilib>:"Draw Multiple Lines.vi"("picture"=w415, "line endpoints"=w408, "color(black)"=w406, "pen"=w410) -> ("new picture"=w414:picture)  [unwired: 5 in]
                n159 = call <vilib>:"Draw Multiple Lines.vi"("picture"=w414, "line endpoints"=w413, "color(black)"=w407, "pen"=w410) -> ("new picture"=w412:picture)  [unwired: 5 in]
                n160 = call <vilib>:"Draw Multiple Lines.vi"("picture"=w412, "line endpoints"=w409, "color(black)"=w405, "pen"=w410) -> ("new picture"=w411:picture)  [unwired: 5 in]
              }
              frame True {
              }
            }
            n161 = Array Size(array=w378) -> (size(s)=w399:i32)
            n162 = Array Size(array=w390) -> (size(s)=w392:i32)
            n163 = Decrement(x=w399) -> (x-1=w396:i32)
            n164 = Decrement(x=w392) -> (x-1=w394:i32)
            n165 = Delete From Array(array=w378, length=1, index=w396) -> (deleted portion=w395:cluster{"x":dbl, "y":dbl}[])  [unwired: 1 out]
            n166 = Delete From Array(array=w390, length=1, index=w394) -> (deleted portion=w391:dbl[])  [unwired: 1 out]
          }
          frame "Bezier" {
            n167 = for {
              tunnel: w457 -> [w476] mode=indexing
              tunnel: [w475] -> w442 mode=indexing
              tunnel: [w472] -> w444 mode=indexing
              tunnel: w440 -> [w471] mode=indexing
              tunnel: [w470] -> w439 mode=indexing
              n168 = Unbundle(w471) -> ("V"=w470:dbl)  [unwired: 2 out]
              n169 = Unbundle(w476) -> ("x"=w474:dbl, "y"=w473:dbl, "th"=w472:dbl)
              n170 = Bundle("x"=w474, "y"=w473) -> (w475:cluster{"x":dbl, "y":dbl})  [unwired: 1 in]
            }
            n171 = Build Array (concatenate)(w453, w442) -> (w441:cluster{"x":dbl, "y":dbl}[])
            n172 = Build Array (concatenate)(w443, w444) -> (w445:dbl[])
            n173 = call "Map Poly to Pixels.vi"("Draw Area Size"=w456, "Position"=w455, "Coords"=w441) -> ("Coords"=w438:cluster{"Horizontal":dbl, "Vertical":dbl}[])  [unwired: 8 in]
            n174 = for {
              tunnel: w438 -> [w464]
              tunnel: w435 -> [w467]
              shift-right: [w458] -> w436
              shift-left: w437 -> [w466]
              tunnel: w434 -> [w461]
              tunnel: w439 -> [_] mode=indexing
              i -> [w462]
              n175 = Array Subset(array=w464, index=w462, length=2) -> (w460:cluster{"Horizontal":dbl, "Vertical":dbl}[])
              n176 = Greater?(x=w462, y=w461) -> (0:w459:bool)
              n177 = Select(t=u32 16711680 ("color(black)"), s=w459, f=u32 6618880 ("color(black)")) -> (s? t:f=w468:u32)
              n178 = call <vilib>:"Draw Multiple Lines.vi"("picture"=w466, "line endpoints"=w460, "color(black)"=w468, "pen"=w467) -> ("new picture"=w458:picture)  [unwired: 5 in]
            }
            n179 = Array Size(array=w441) -> (size(s)=w454:i32)
            n180 = Array Size(array=w445) -> (size(s)=w447:i32)
            n181 = Decrement(x=w454) -> (x-1=w451:i32)
            n182 = Decrement(x=w447) -> (x-1=w449:i32)
            n183 = Delete From Array(array=w441, length=1, index=w451) -> (deleted portion=w450:cluster{"x":dbl, "y":dbl}[])  [unwired: 1 out]
            n184 = Delete From Array(array=w445, length=1, index=w449) -> (deleted portion=w446:dbl[])  [unwired: 1 out]
          }
          frame "Circle" {
            # "Connect for accel and decel"
            n185 = for {
              tunnel: w504 -> [w535] mode=indexing
              tunnel: [w534] -> w486 mode=indexing
              tunnel: [w531] -> w490 mode=indexing
              tunnel: w483 -> [w530] mode=indexing
              tunnel: [w529] -> w481 mode=indexing
              n186 = Unbundle(w530) -> ("V"=w529:dbl)  [unwired: 2 out]
              n187 = Unbundle(w535) -> ("x"=w533:dbl, "y"=w532:dbl, "th"=w531:dbl)
              n188 = Bundle("x"=w533, "y"=w532) -> (w534:cluster{"x":dbl, "y":dbl})  [unwired: 1 in]
            }
            n189 = Build Array (concatenate)(w499, w486) -> (w485:cluster{"x":dbl, "y":dbl}[])
            n190 = Build Array (concatenate)(w489, w490) -> (w491:dbl[])
            n191 = call "Map Poly to Pixels.vi"("Draw Area Size"=w503, "Position"=w501, "Coords"=w485) -> ("Coords"=w482:cluster{"Horizontal":dbl, "Vertical":dbl}[])  [unwired: 8 in]
            n192 = for {
              tunnel: w482 -> [w513] mode=indexing
              tunnel: w481 -> [w512] mode=indexing
              shift-right: [w512] -> _
              shift-left: -inf -> [w516]
              tunnel: [w513] -> w479 mode=indexing if=w507
              tunnel: [w513] -> w478 mode=indexing if=w506
              tunnel: [w513] -> w477 mode=indexing if=w505
              n193 = Subtract(x=w512, y=w516) -> (x-y=w510:dbl)
              n194 = Absolute Value(x=w510) -> (abs(x)=w515:dbl)
              n195 = Less?(x=w515, y=1e-05) -> (x < y?=w507:bool)
              n196 = Greater Than 0?(x=w510) -> (x > 0?=w511:bool)
              n197 = Less Than 0?(x=w510) -> (x < 0?=w509:bool)
              n198 = Not(x=w507) -> (.not. x?=w508:bool)
              n199 = And(x=w508, y=w511) -> (x .and. y?=w506:bool)
              n200 = And(x=w508, y=w509) -> (x .and. y?=w505:bool)
            }
            n201 = case shown="False" w484 {
              tunnel: w502 -> [w527 w528]
              tunnel: [w524 w528] -> w488
              tunnel: w487 -> [w523 _]
              tunnel: w479 -> [w520 _]
              tunnel: w478 -> [w519 _]
              tunnel: w477 -> [w518 _]
              frame False {
                n202 = call <vilib>:"Draw Multiple Lines.vi"("picture"=w527, "line endpoints"=w520, "color(black)"=u32 13055, "pen"=w523) -> ("new picture"=w526:picture)  [unwired: 5 in]
                n203 = call <vilib>:"Draw Multiple Lines.vi"("picture"=w526, "line endpoints"=w519, "color(black)"=u32 6618880, "pen"=w523) -> ("new picture"=w525:picture)  [unwired: 5 in]
                n204 = call <vilib>:"Draw Multiple Lines.vi"("picture"=w525, "line endpoints"=w518, "color(black)"=u32 16747538, "pen"=w523) -> ("new picture"=w524:picture)  [unwired: 5 in]
              }
              frame True {
              }
            }
            n205 = Array Size(array=w485) -> (size(s)=w500:i32)
            n206 = Array Size(array=w491) -> (size(s)=w493:i32)
            n207 = Decrement(x=w500) -> (x-1=w497:i32)
            n208 = Decrement(x=w493) -> (x-1=w495:i32)
            n209 = Delete From Array(array=w485, length=1, index=w497) -> (deleted portion=w496:cluster{"x":dbl, "y":dbl}[])  [unwired: 1 out]
            n210 = Delete From Array(array=w491, length=1, index=w495) -> (deleted portion=w492:dbl[])  [unwired: 1 out]
          }
        }
      }
      n211 = Array Size(array=w334) -> (size(s)=w333:i32)
      n212 = Decrement(x=w333) -> (x-1=w332:i32)
      n213 = In Range and Coerce(upper limit=w332, x=w325, lower limit=u16 0 ("Width")) -> (coerced(x)=w330:i32)  [unwired: 1 out]
      n214 = Index Array(array=w335, index=w330) -> (element=w336:dbl)
      n215 = Index Array(array=w334, index=w330) -> (element=w339:cluster{"x":dbl, "y":dbl})
      n216 = Unbundle(w339) -> ("x"=w338:dbl, "y"=w337:dbl)
      n217 = Bundle("x"=w338, "y"=w337, "th"=w336) -> (w324:cluster{"x":dbl, "y":dbl, "th":dbl})  [unwired: 1 in]
    }
  }
  "new picture" <- w10
  "Path Points" <- w9
  "Path Points MEGA" <- w3
  "Output Point" <- w2
